vi "Thermometer analysis for loop.vi"() -> ()   [LabVIEW 2020]
uses:
  <vilib>/Analysis/baseanly.llb/Mean (DBL).vi
  <vilib>/Analysis/NI_AALBase.lvlib
panel:
  out "T-AVE":dbl
  out "T-MIN":dbl
  out "T-MAX":dbl
  out "Waveform Graph":dbl[](graph)
  out "Waveform Chart":dbl(graph)
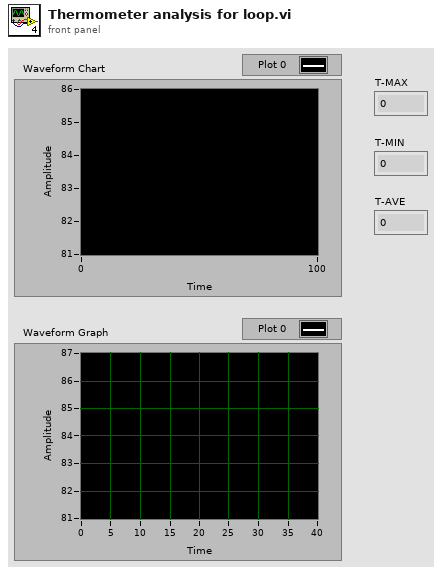
[diagram p1: front panel]
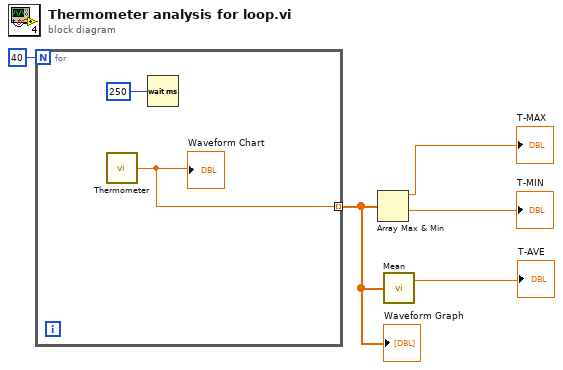
[diagram p0: block diagram]
diagram:
  n1 = for {
    N: 40 -> [_]
    tunnel: [w6] -> w1 mode=indexing
    n2 = call "Thermometer.vi"() -> ("Temperature (deg F)"=w6:dbl)  [unwired: 1 in]
    "Waveform Chart" <- w6
    n3 = Wait (ms)(milliseconds to wait=u32 250 ("millisecond timer value")) -> ()  [unwired: 1 out]
  }
  "Waveform Graph" <- w1
  n4 = Array Max & Min(array=w1) -> (max value=→"T-MAX":dbl, min value=→"T-MIN":dbl)  [unwired: 2 out]
  n5 = call-poly <vilib>:"Mean.vi"("X"=w1) -> ("mean"=→"T-AVE":dbl)  [unwired: 1 out]
